vi "SetAttribute.vi"(8 "error in (no error)":errorcluster, 10 "Set Attribute":T1, 11 "Data_AllInOne in":refnum<class "Data_AllInOne.lvclass">) -> (0 "error out":errorcluster, 3 "Data_AllInOne out":refnum<class "Data_AllInOne.lvclass">)   [LabVIEW 2020, in "Data_AllInOne.lvclass"]
uses:
  Data_AllInOne.lvclass
  Attribute.vi
  Data_AllInOne.lvclass/Data_AllInOne.ctl
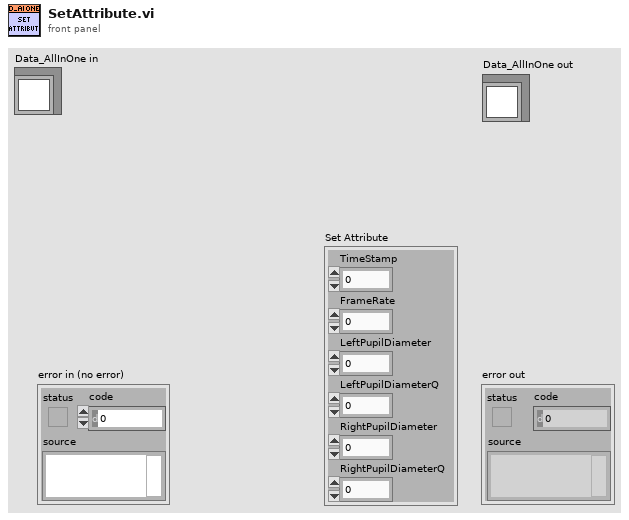
[diagram p1: front panel]
types:
  T1 = typedef "Data_AllInOne.lvclass/Attribute.vi" = cluster{"TimeStamp":u64, "FrameRate":dbl, "LeftPupilDiameter":dbl, "LeftPupilDiameterQ":dbl, "RightPupilDiameter":dbl, "RightPupilDiameterQ":dbl}
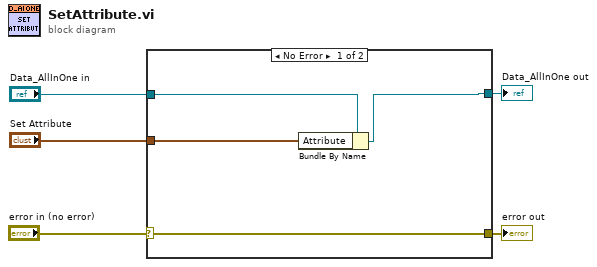
[diagram p0: block diagram]
diagram:
  n1 = case shown="No Error" "error in (no error)" {
    selector: "error in (no error)" -> [w9 w11]
    tunnel: [w9 w11] -> w4
    tunnel: [w7 w10] -> w3
    tunnel: "Data_AllInOne in" -> [w8 w10]
    tunnel: "Set Attribute" -> [w6 _]
    frame No Error {
      n2 = Bundle By Name(cluster=w8, "Attribute"=w6) -> (w7:refnum<class "Data_AllInOne.lvclass">)
    }
    frame Error {
    }
  }
  "error out" <- w4
  "Data_AllInOne out" <- w3
